vi "GetMostRecentExperimentRun.vi"(11 "Experiment":T6={"File Path"=path "", "Operator"="", "Project"="", "Target Dose (dpa)"=0.0, "Sample"={"Name"="", "Description"="", "Molar Mass (g/mol)"=0.0, "Density (g/cm^3)"=0.0, "Irradiation Area (cm^2)"=0.0, "SRIM Damage Peak (disp * ions/cm)"=0.0}, "Beam Line"={"Type"=enum."Ion Beam Analysis", "Ion"=enum."H", "Charge State"=0, "Total Source Ion Energy (kV)"=nan}, "Runs"=[]} {"Beam Line"."Charge State" min=1}) -> (3 "Recent Experiment Run":T1)   [LabVIEW 2012]
uses:
  Experiment.ctl
  Sample.ctl
  BeamLine.ctl
  BeamLineType.ctl
  BeamLineIon.ctl
  ExperimentRun.ctl
  ExperimentRunTiming.ctl
  ExperimentRunDose.ctl
  ExperimentRunFluence.ctl
  ExperimentRunTotalCharge.ctl
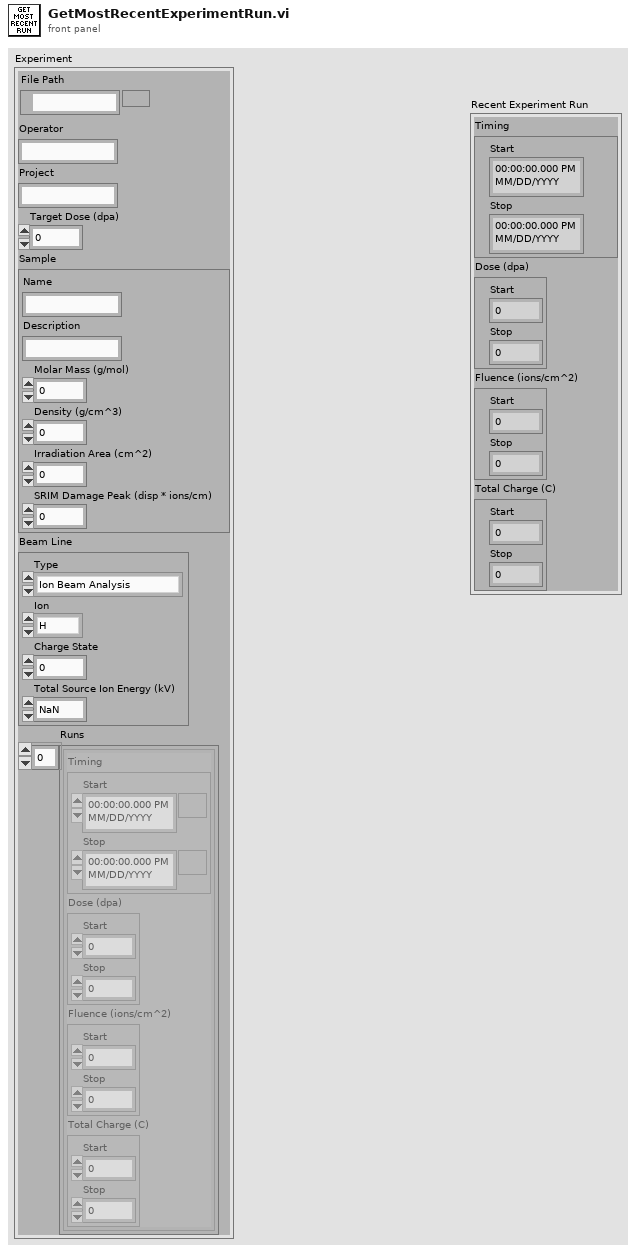
[diagram p1: front panel]
types:
  T1 = typedef "ExperimentRun.ctl" = cluster{"Timing":T2, "Dose (dpa)":T3, "Fluence (ions/cm^2)":T4, "Total Charge (C)":T5}
  T2 = typedef "ExperimentRunTiming.ctl" = cluster{"Start":timestamp, "Stop":timestamp}
  T3 = typedef "ExperimentRunDose.ctl" = cluster{"Start":dbl, "Stop":dbl}
  T4 = typedef "ExperimentRunFluence.ctl" = cluster{"Start":dbl, "Stop":dbl}
  T5 = typedef "ExperimentRunTotalCharge.ctl" = cluster{"Start":dbl, "Stop":dbl}
  T6 = typedef "Experiment.ctl" = cluster{"File Path":path, "Operator":string, "Project":string, "Target Dose (dpa)":dbl, "Sample":T7, "Beam Line":T8, "Runs":T1[]}
  T7 = typedef "Sample.ctl" = cluster{"Name":string, "Description":string, "Molar Mass (g/mol)":dbl, "Density (g/cm^3)":dbl, "Irradiation Area (cm^2)":dbl, "SRIM Damage Peak (disp * ions/cm)":dbl}
  T8 = typedef "BeamLine.ctl" = cluster{"Type":T9, "Ion":T10, "Charge State":u8, "Total Source Ion Energy (kV)":dbl}
  T9 = typedef "BeamLineType.ctl" = enum16{"Ion Beam Analysis", "Auxiliary", "Radiation Damage"}
  T10 = typedef "BeamLineIon.ctl" = enum16{"H", "He", "C", "Fe", "Ni", "Pt", "Si", "Ag", "Au"}
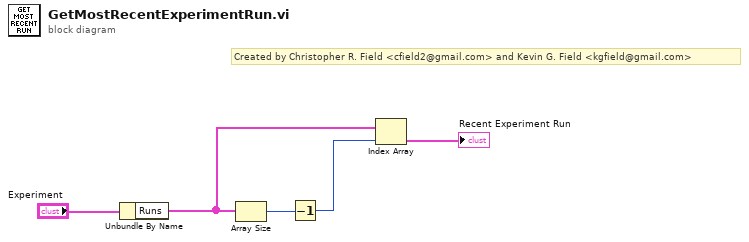
[diagram p0: block diagram]
diagram:
  # "Created by Christopher R. Field <cfield2@gmail.com> and Kevin G. Field <kgfield@gmail.com>"
  n1 = Unbundle By Name("Experiment") -> ("Runs"=w3:T1[])
  n2 = Array Size(array=w3) -> (size(s)=w4:i32)
  n3 = Decrement(x=w4) -> (x-1=w2:i32)
  n4 = Index Array(array=w3, index=w2) -> (element=→"Recent Experiment Run":T1)
